vi "Ins2Pos.vi"(1 "Ins":i16[](array[numeric])) -> (0 "Pos":dbl)   [LabVIEW 2016]
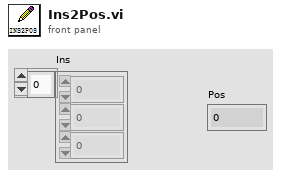
[diagram p1: front panel]
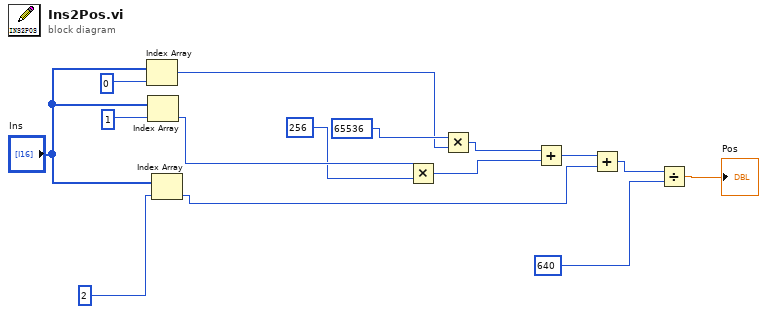
[diagram p0: block diagram]
diagram:
  n1 = Index Array(array="Ins", index=0) -> (element=w7:i16)
  n2 = Index Array(array="Ins", index=1) -> (element=w5:i16)
  n3 = Index Array(array="Ins", index=2) -> (element=w3:i16)
  n4 = Multiply(x=w5, y=256) -> (x*y=w13:i32)
  n5 = Multiply(x=65536, y=w7) -> (x*y=w14:i32)
  n6 = Add(x=w14, y=w13) -> (x+y=w12:i32)
  n7 = Add(x=w12, y=w3) -> (x+y=w11:i32)
  n8 = Divide(x=w11, y=640) -> (x/y=→"Pos":dbl)
